vi "TI sbRIO Main (FPGA).vi"() -> ()   [LabVIEW 2013]
uses:
  Type Defs/Controller Names.ctl
  <vilib>/Platform/TimedLoop/XDataNode/timing_clust.ctl
  <vilib>/Platform/TimedLoop/XDataNode/nitl_modes.ctl
  <vilib>/Platform/TimedLoop/XDataNode/wakeup.ctl
  <vilib>/rvi/FXPMathLib/basic elements/FxpIntAccumulator/subVIs/nifxpmath_IntAccumulator_SimConfig.ctl
  <vilib>/rvi/FXPMathLib/FxpSqrt/subVIs/nifxpmath_Sqrt_SimConfig.ctl
  <vilib>/fxp/LVFixedPointOverflowPolicyTypeDef.ctl
  <vilib>/rvi/FXPMathLib/FxpDiv/subVIs/nifxpmath_Div_SimConfig.ctl
  <vilib>/rvi/Emulation/niFpgaSctlEmulationGetInTimedLoop.vi
  <vilib>/rvi/Emulation/niFpgaEmulationReportErrorSimple.vi
  <vilib>/rvi/Emulation/niFpgaGetClockAttributes.vi
  <vilib>/rvi/eio/common/nirviEmuTemplateMethod_errors.vi
  <vilib>/rvi/Emulation/niFpgaCriticalErrorInLSC.vi
  <vilib>/rvi/Analysis/common/codeGenErrors/XNode/niFpgaXNodeCodeGenErrorHandle.vi
  <vilib>/rvi/FXPMathLib/basic elements/FxpIntAccumulator/simVIs/DllFxpIntAccumulator_sub.vi
  <vilib>/rvi/Analysis/utilities/niFPGA Threshold Crossing Logic.vi
  <vilib>/rvi/FXPMathLib/FxpSqrt/simVIs/DllSqrtTemp_sub.vi
  <vilib>/rvi/FXPMathLib/FxpDiv/simVIs/DllFxpDivTemp_sub.vi
  <vilib>/eio/EIONode/EIONode.xnode
  <vilib>/rvi/FXPMathLib/FxpMul/XNode/nifxpmath_Multiplier.xnode
  <vilib>/rvi/FXPMathLib/FxpAdd/XNode/nifxpmath_Add.xnode
  <vilib>/rvi/FXPMathLib/FxpSub/XNode/nifxpmath_Sub.xnode
  <vilib>/rvi/Analysis/measure/period/templates/niFPGA Period Edge Direction.ctl
  <vilib>/rvi/Analysis/measure/mean-var-std/XNode/niFpgaMean-Var-Std.xnode
  <vilib>/Platform/TimedLoop/XDataNode/XDataNode.xnode
  <vilib>/rvi/FXPMathLib/basic elements/FxpIntAccumulator/XNode/nifxpmath_IntAccumulator.xnode
  <vilib>/rvi/Analysis/measure/period/XNode/niFpgaAnalogPeriod.xnode
  <vilib>/rvi/Analysis/measure/dc-rms/XNode/niFpgaDC-RMS.xnode
  <vilib>/rvi/FXPMathLib/FxpSqrt/XNode/nifxpmath_Sqrt.xnode
  <vilib>/rvi/FXPMathLib/FxpDiv/XNode/nifxpmath_Div.xnode
  <vilib>/rvi/FXPMathLib/sim/FxpSim.dll
  <vilib>/Platform/TimedLoop/XDataNode/XDNodeRunTimeDep.lvlib
  <vilib>/rvi/DataTransferAndStorage/Container/XNode/niFpgaContainer.xnode
  <vilib>/rvi/FIFO/Fifo_Resource/niFpgaFifoEmulationRefIn.vi
panel:
  out "Spare_3":fxp<+/-,20,12>
  out "Spare_1":fxp<+/-,20,12>
  in  "Mod1 On?":bool
  in  "Mod2 On?":bool
  in  "Mod2 Pulsing?":bool
  in  "Mod3 Pulsing?":bool
  in  "Mod1 Pulsing?":bool
  in  "Mod3 On?":bool
  in  "Module 3 Pulse Duty":i16
  in  "Module 2 Pulse Duty":i16
  in  "Module 1 Pulse Duty":i16
  in  "Pulse Frequency":sgl=20.0
  in  "Controller Type:":T1
  in  "InvertPWM":bool
  in  "Conti Window":i32=434
  out "Temp 2":fxp<+/-,16,8> format="%#.1f"
  out "Currents (RMS)":fxp<+,26,7>[](array[numeric])
  out "Speed (RPM)":fxp<+,32,18>[](array[numeric])
  in  "Spike Window":i32=125
  in  "Min Window":i32=125
  in  "Max Window":i32=125
  in  "Disarm Level":i32=125
  in  "Arm Level":i32=125
  in  "PS Control":bool=TRUE
  out "Temp":fxp<+/-,16,8> format="%#.1f"
  in  "AO3":fxp<+/-,20,5>
  in  "AO2":fxp<+/-,20,5>
  in  "AO1":fxp<+/-,20,5>
  in  "AO0":fxp<+/-,20,5>
  in  "Kuhnke Window":i32=125
  in  "Speed Hysteresis":fxp<+,23,5>=1.0
  in  "Current Offset":fxp<+/-,18,7>=-60.09521484375 format="%#_14g"
  in  "Current Scale":fxp<+,16,5>=24.0380859375 format="%#_13g"
  out "Actual Loop Time":u32
  in  "Loop Timer (uSec)":u32=100
  in  "Current Offsets":fxp<+/-,24,7>[](array[numeric])=[0.0, 0.0, 0.0, 0.0, 0.0, 0.0]
  out "Elapsed Times":u64[](array[numeric])
  in  "Timer Resets":bool[](array[boolean])=[FALSE, FALSE, FALSE, FALSE, FALSE, FALSE]
  in  "Threshold":fxp<+/-,24,6>=1.0
  in  "Consec Samples":i32=125
  out "Actual Pump Starts":u32[](array[numeric])
  in  "Reset":bool
  in  "Duty (Ticks) 6":i32
  in  "Duty (Ticks) 5":i32
  in  "Duty (Ticks) 4":i32
  in  "Duty (Ticks) 3":i32
  in  "PWM Period (Ticks)":u32=40000000
  in  "Duty (Ticks) 1":i32
  in  "Duty (Ticks) 2":i32
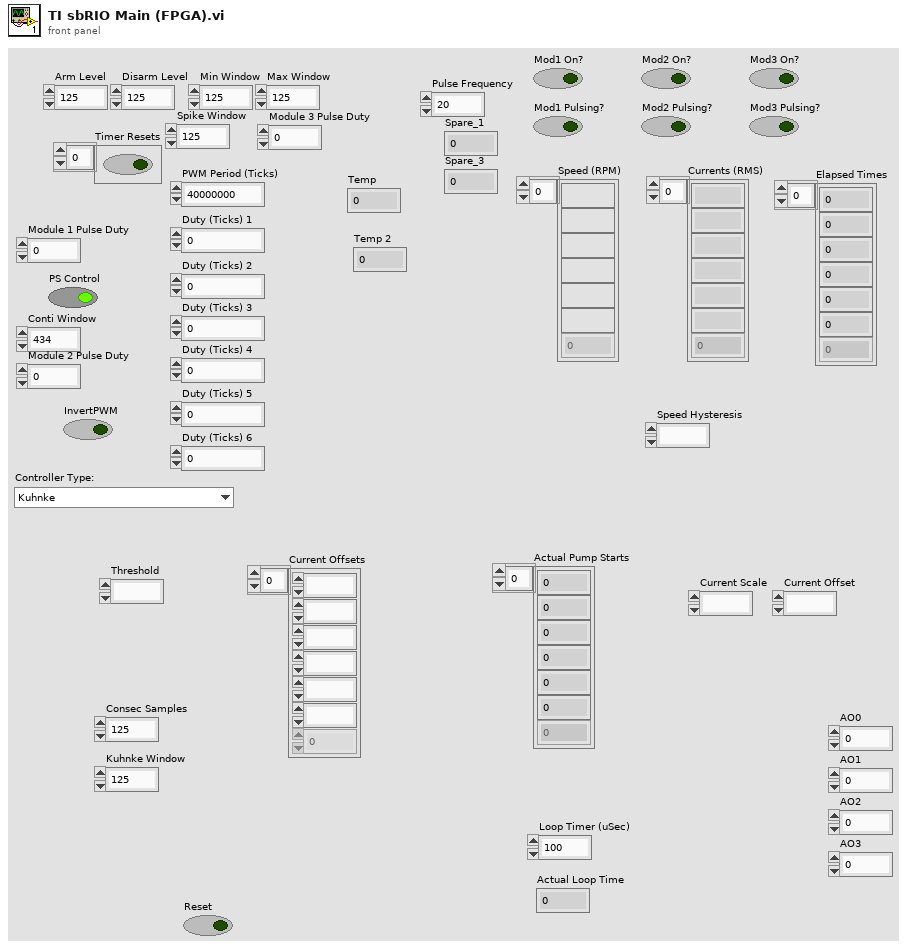
[diagram p1: front panel]
types:
  T1 = typedef "Controller Names.ctl" = enum16{"Kuhnke", "Conti", "Helbako", "TI PWM", "PSA", "Hella Gas", "Hella Diesel", "8 Comm", "10 Comm", "8 Comm Hella", "10 Comm Hella", "8 Comm Omron", "10 Comm Omron", "8 Comm Nissan", "10 Comm Nissan"}
  T2 = typedef "XDNodeRunTimeDep.lvlib/timing_clust.ctl" = cluster{"Expected End [f-1]":u64, "Actual End [f-1]":u64, "Finished Late? [f-1]":bool, "Expected End [i-1]":u64, "Actual End [i-1]":u64, "Finished Late? [i-1]":bool, "Expected Start [i]":u64, "Actual Start [i]":u64, "Expected Start [f]":u64, "Actual Start [f]":u64, "Source Name":string, "Structure Name":string, "Period":i64, "Deadline":i64, "Offset":i64, "Start":i64, "Priority":i32, "Timeout":i32, "Mode":T3, "Wakeup Reason":T4, "Error":errorcluster, "Source Type":string, "Secondary Source Type":string, "Global End Time":u64, "Global Start Time":u64, "Frame Duration":u64, "Iteration Duration":u64, "Assigned CPU":i32, "I/O Scan Engine Mode":u32}
  T3 = typedef "XDNodeRunTimeDep.lvlib/nitl_modes.ctl" = enum32{"No Change", "Process missed periods, maintain original phase", "Discard missed periods, maintain original phase", "Process missed periods, ignore original phase", "Discard missed periods, ignore original phase"}
  T4 = typedef "XDNodeRunTimeDep.lvlib/wakeup.ctl" = enum32{"Normal", "Aborted", "Asynchronous wakeup", "Timing source error", "Timed loop error", "Timeout"}
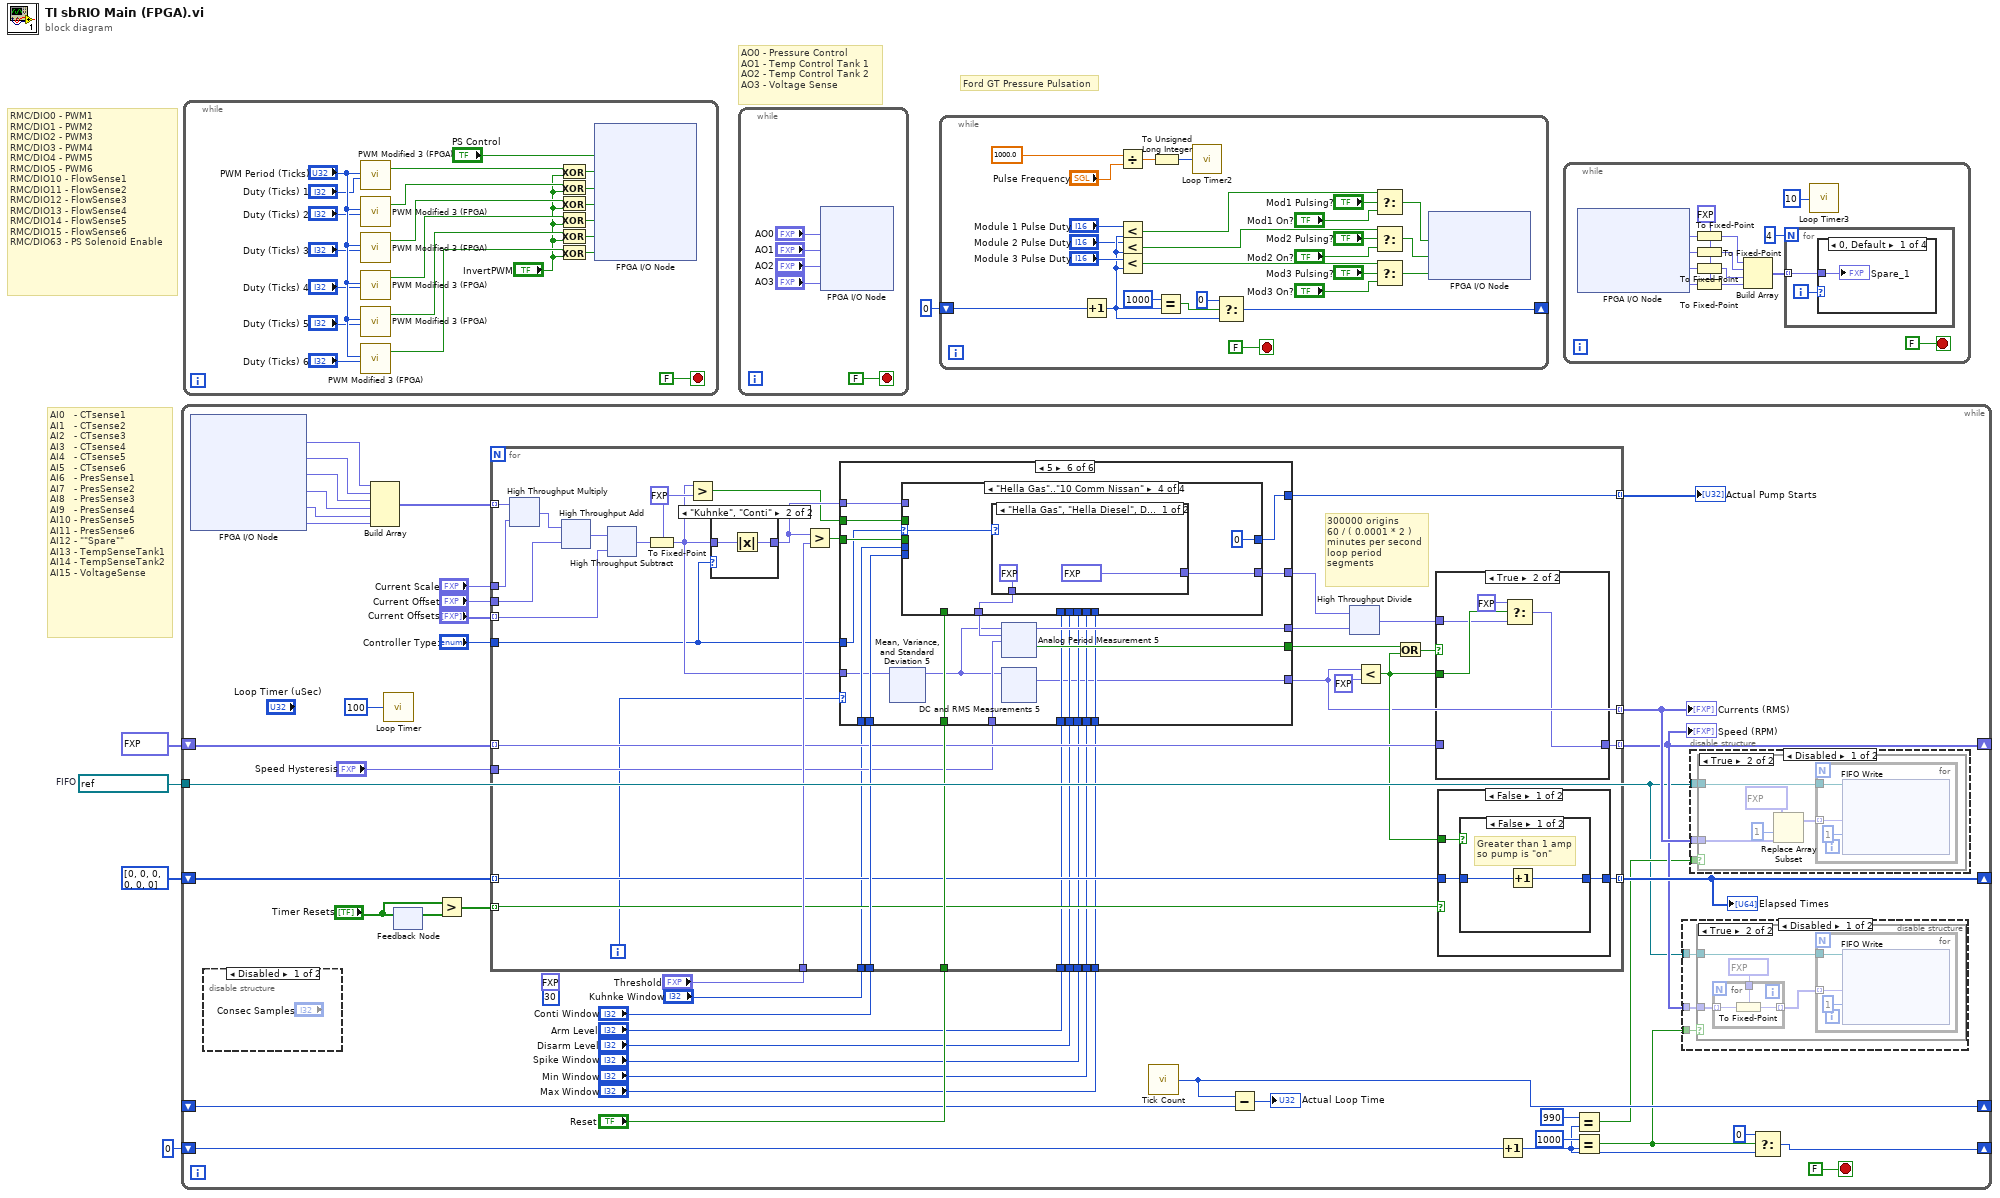
[diagram p0: block diagram]
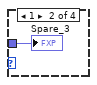
[diagram p2: hidden frame]
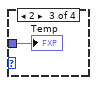
[diagram p3: hidden frame]
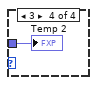
[diagram p4: hidden frame]
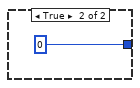
[diagram p12: hidden frame]
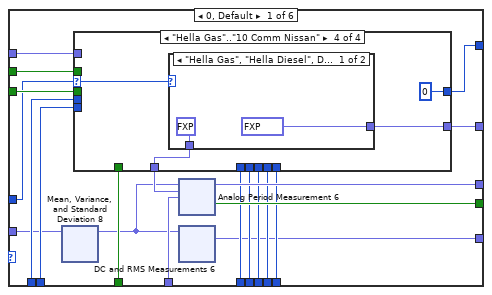
[diagram p14: hidden frame]
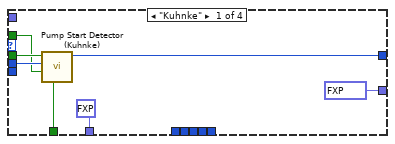
[diagram p15: hidden frame]
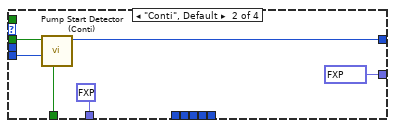
[diagram p16: hidden frame]
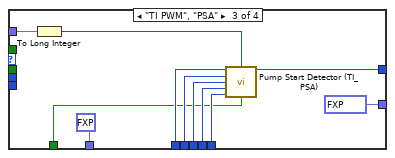
[diagram p17: hidden frame]
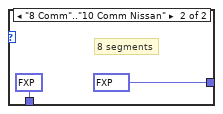
[diagram p18: hidden frame]
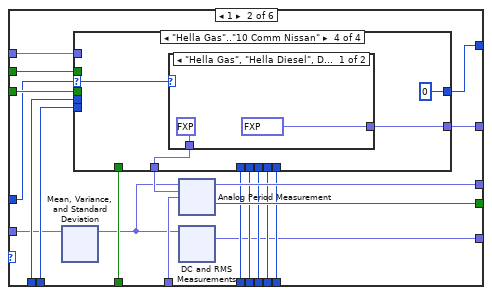
[diagram p19: hidden frame]
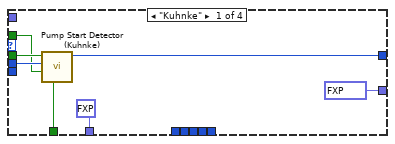
[diagram p20: hidden frame]
diagram:
  w2 = refnum<k21> "Current FIFO"  # FIFO
  # "Ford GT Pressure Pulsation"
  # "RMC/DIO0 - PWM1\nRMC/DIO1 - PWM2\nRMC/DIO2 - PWM3\nRMC/DIO3 - PWM4\nRMC/DIO4 - PWM5\nRMC/DIO5 - PWM6\nRMC/DIO10 - FlowSense1\nRMC/DIO11 - FlowSense2\nRMC/DIO12 - FlowSense3\nRMC/DIO13 - FlowSense4\nRMC/DIO14 - FlowSense5\nRMC/DIO15 - FlowSense6\nRMC/DIO63 - PS Solenoid Enable"
  # "AO0 - Pressure Control\nAO1 - Temp Control Tank 1\nAO2 - Temp Control Tank 2\nAO3 - Voltage Sense"
  # "AI0   - CTsense1\nAI1   - CTsense2\nAI2   - CTsense3\nAI3   - CTsense4\nAI4   - CTsense5\nAI5   - CTsense6\nAI6   - PresSense1\nAI7   - PresSense2\nAI8   - PresSense3\nAI9   - PresSense4\nAI10 - PresSense5\nAI11 - PresSense6\nAI12 - \"\"Spare\"\"\nAI13 - TempSenseTank1\nAI14 - TempSenseTank2\nAI15 - VoltageSense"
  n1 = while {
    shift-right: [w10] -> _
    shift-left: fxp<+,32,18>[] [0.0, 0.0, 0.0, 0.0, 0.0, 0.0] -> [w45]
    shift-right: [w43] -> _
    shift-left: u64[] [0, 0, 0, 0, 0, 0] -> [w44]
    shift-right: [w38] -> _
    shift-left: _ -> [w37]
    shift-right: [w14] -> _
    shift-left: u32 0 ("Tick Count(uSec)") -> [w17]
    tunnel: w2 -> [w7]
    stop <- FALSE stop-if-true
    (unwired) fxp<+/-,24,6> 1.0 ("Threshold")
    (unwired) 30 ("Kuhnke Window")
    n2 = xnode "FPGA I/O Node"() -> ("Current 1 (AI0)"=w28:fxp<+/-,24,5>, "Current 2 (AI1)"=w49:fxp<+/-,24,5>, "Current 3 (AI2)"=w32:fxp<+/-,24,5>, "Current 4 (AI3)"=w31:fxp<+/-,24,5>, "Current 5 (AI4)"=w30:fxp<+/-,24,5>, "Current 6 (AI5)"=w29:fxp<+/-,24,5>)  [unwired: 6 in, 6 out]
    n3 = disable-structure shown="Disabled" {
      frame Disabled {
      }
      frame Enabled {
      }
    }
    n4 = Build Array(w28, w49, w32, w31, w30, w29) -> (w46:fxp<+/-,24,5>[])
    n5 = call "Loop Timer"("Count(uSec)"=u32 100 ("Loop Timer (uSec)")) -> ()  [unwired: 1 out]
    n6 = feedback-in #1("Timer Resets") -> ()
    n7 = feedback #1() -> (w41:bool[])  [unwired: 1 in]
    n8 = Greater?(x="Timer Resets", y=w41) -> (0:w40:bool[])
    n9 = for {
      tunnel: "Conti Window" -> [w111]
      tunnel: [w110] -> w27 mode=indexing
      tunnel: "Threshold" -> [w109]
      tunnel: "Reset" -> [w107]
      tunnel: w46 -> [w91] mode=indexing
      tunnel: w44 -> [w98] mode=indexing
      tunnel: [w97] -> w43 mode=indexing
      tunnel: w45 -> [w102] mode=indexing
      tunnel: [w101] -> w10 mode=indexing
      tunnel: w40 -> [w96] mode=indexing
      tunnel: "Current Offsets" -> [w88] mode=indexing
      tunnel: [w76] -> w13 mode=indexing
      tunnel: "Current Scale" -> [w90]
      tunnel: "Current Offset" -> [w89]
      tunnel: "Speed Hysteresis" -> [w95]
      tunnel: "Kuhnke Window" -> [w94]
      tunnel: "Arm Level" -> [w85]
      tunnel: "Disarm Level" -> [w84]
      tunnel: "Spike Window" -> [w83]
      tunnel: "Min Window" -> [w82]
      tunnel: "Max Window" -> [w81]
      tunnel: "Controller Type:" -> [w74]
      i -> [w77]
      w79 = fxp<+/-,26,7> 0.0 ("out")
      # "300000 origins\n60 / ( 0.0001 * 2 )\nminutes per second\nloop period\nsegments"
      n10 = xnode ("High Throughput Multiply")("x"=w91, "y"=w90) -> ("x*y"=w92:fxp<+/-,40,10>)
      n11 = xnode ("High Throughput Add")("x"=w92, "y"=w89) -> ("x+y"=w80:fxp<+/-,41,11>)
      n12 = xnode "High Throughput Subtract"("x"=w80, "y"=w88) -> ("x-y"=w93:fxp<+/-,42,12>)
      n13 = To Fixed-Point(fixed-point type=w79, number=w93) -> (fixed-point=w75:fxp<+/-,26,7>)
      n14 = Greater?(x=w75, y=w79) -> (0:w78:bool)
      n15 = case shown="\"Kuhnke\", \"Conti\"" w74 {
        tunnel: w75 -> [w112 w113]
        tunnel: [w112 w114] -> w87
        frame Default {
        }
        frame "Kuhnke", "Conti" {
          n16 = Absolute Value(x=w113) -> (abs(x)=w114:fxp<+,26,7>)
        }
      }
      n17 = Greater?(x=w87, y=w109) -> (0:w108:bool)
      n18 = case shown="5" w77 {
        tunnel: w108 -> [w174 w526 w878 w1230 w1582 w1934]
        tunnel: w111 -> [w173 w525 w877 w1229 w1581 w1933]
        tunnel: [w172 w524 w876 w1228 w1580 w1932] -> w110
        tunnel: w107 -> [w166 w518 w870 w1222 w1574 w1926]
        tunnel: w75 -> [w155 w507 w859 w1211 w1563 w1915]
        tunnel: [w157 w509 w861 w1213 w1565 w1917] -> w76
        tunnel: [w171 w523 w875 w1227 w1579 w1931] -> w103
        tunnel: [w170 w522 w874 w1226 w1578 w1930] -> w100
        tunnel: w74 -> [w169 w521 w873 w1225 w1577 w1929]
        tunnel: w95 -> [w168 w520 w872 w1224 w1576 w1928]
        tunnel: w94 -> [w167 w519 w871 w1223 w1575 w1927]
        tunnel: w87 -> [w165 w517 w869 w1221 w1573 w1925]
        tunnel: [w164 w516 w868 w1220 w1572 w1924] -> w86
        tunnel: w85 -> [w163 w515 w867 w1219 w1571 w1923]
        tunnel: w84 -> [w162 w514 w866 w1218 w1570 w1922]
        tunnel: w83 -> [w161 w513 w865 w1217 w1569 w1921]
        tunnel: w82 -> [w160 w512 w864 w1216 w1568 w1920]
        tunnel: w81 -> [w159 w511 w863 w1215 w1567 w1919]
        tunnel: w78 -> [w158 w510 w862 w1214 w1566 w1918]
        frame 0, Default {
          n19 = xnode ("Mean, Variance, and Standard Deviation 8")("input data"=w155) -> ("mean"=w154:fxp<+/-,26,7>)  [unwired: 1 in, 1 out]
          n20 = case shown="\"Hella Gas\"..\"10 Comm Nissan\"" w169 {
            selector: w169 -> [_ _ _ w277]
            tunnel: w174 -> [w256 w263 _ _]
            tunnel: w173 -> [_ w262 _ _]
            tunnel: [w255 w261 w267 u32 0 ("Restarts")] -> w172
            tunnel: w166 -> [w257 w260 w265 _]
            tunnel: w167 -> [w254 _ _ _]
            tunnel: w165 -> [_ _ w274 _]
            tunnel: [fxp<+,32,19> 300000.0 ("x") fxp<+,32,19> 300000.0 ("x") fxp<+,32,19> 300000.0 ("x") w276] -> w164
            tunnel: w163 -> [_ _ w272 _]
            tunnel: w162 -> [_ _ w271 _]
            tunnel: w161 -> [_ _ w270 _]
            tunnel: w160 -> [_ _ w269 _]
            tunnel: w159 -> [_ _ w268 _]
            tunnel: w158 -> [w252 _ _ _]
            tunnel: [fxp<+/-,24,7> 0.0 ("threshold level") fxp<+/-,24,7> 0.0 ("threshold level") fxp<+/-,24,7> 0.0 ("threshold level") w275] -> w156
            frame "Kuhnke" {
              n21 = call "Pump Start Detector (Kuhnke).vi"("Reset"=w257, "Pos?"=w252, "Window"=w254, "Pos Cross"=w256) -> ("Starts"=w255:u32)  [unwired: 6 in, 1 out]
            }
            frame "Conti", Default {
              n22 = call "Pump Start Detector (Conti).vi"("Reset"=w260, "Consec Samples"=w262, "Crossing?"=w263) -> ("Restarts"=w261:u32)  [unwired: 8 in]
            }
            frame "TI PWM", "PSA" {
              n23 = To Long Integer(number=w274) -> (32bit integer=w266:i32)
              n24 = call "Pump Start Detector (TI_PSA).vi"("Arm Level"=w272, "Level"=w266, "Disarm Level"=w271, "Spike Window"=w270, "Min Window"=w269, "Max Window"=w268, "Reset"=w265) -> ("Restarts"=w267:u32)  [unwired: 8 in]
            }
            frame "Hella Gas".."10 Comm Nissan" {
              n25 = case shown="\"Hella Gas\", \"Hella Diesel\", Default" w277 {
                tunnel: [fxp<+,32,19> 300000.0 ("x") fxp<+,32,19> 75000.0 ("x")] -> w276
                tunnel: [fxp<+/-,24,7> 0.0 ("threshold level") fxp<+/-,24,7> 6.75 ("threshold level")] -> w275
                frame "Hella Gas", "Hella Diesel", Default {
                }
                frame "8 Comm".."10 Comm Nissan" {
                  # "8 segments"
                }
              }
            }
          }
          n26 = xnode ("Analog Period Measurement 6")("input data"=w154, "threshold level"=w156, "hysteresis"=w168) -> ("period (samples)"=w170:fxp<+,32,16>, "output valid"=w171:bool)  [unwired: 2 in, 2 out]
          n27 = xnode ("DC and RMS Measurements 6")("input data"=w154) -> ("RMS"=w157:fxp<+,26,7>)  [unwired: 1 in, 1 out]
        }
        frame 1 {
          n28 = xnode ("Mean, Variance, and Standard Deviation")("input data"=w507) -> ("mean"=w506:fxp<+/-,26,7>)  [unwired: 1 in, 1 out]
          n29 = case shown="\"Hella Gas\"..\"10 Comm Nissan\"" w521 {
            selector: w521 -> [_ _ _ w629]
            tunnel: w526 -> [w608 w615 _ _]
            tunnel: w525 -> [_ w614 _ _]
            tunnel: [w607 w613 w619 u32 0 ("Restarts")] -> w524
            tunnel: w518 -> [w609 w612 w617 _]
            tunnel: w519 -> [w606 _ _ _]
            tunnel: w517 -> [_ _ w626 _]
            tunnel: [fxp<+,32,19> 300000.0 ("x") fxp<+,32,19> 300000.0 ("x") fxp<+,32,19> 300000.0 ("x") w628] -> w516
            tunnel: w515 -> [_ _ w624 _]
            tunnel: w514 -> [_ _ w623 _]
            tunnel: w513 -> [_ _ w622 _]
            tunnel: w512 -> [_ _ w621 _]
            tunnel: w511 -> [_ _ w620 _]
            tunnel: w510 -> [w604 _ _ _]
            tunnel: [fxp<+/-,24,7> 0.0 ("threshold level") fxp<+/-,24,7> 0.0 ("threshold level") fxp<+/-,24,7> 0.0 ("threshold level") w627] -> w508
            frame "Kuhnke" {
              n30 = call "Pump Start Detector (Kuhnke).vi"("Reset"=w609, "Pos?"=w604, "Window"=w606, "Pos Cross"=w608) -> ("Starts"=w607:u32)  [unwired: 6 in, 1 out]
            }
            frame "Conti", Default {
              n31 = call "Pump Start Detector (Conti).vi"("Reset"=w612, "Consec Samples"=w614, "Crossing?"=w615) -> ("Restarts"=w613:u32)  [unwired: 8 in]
            }
            frame "TI PWM", "PSA" {
              n32 = To Long Integer(number=w626) -> (32bit integer=w618:i32)
              n33 = call "Pump Start Detector (TI_PSA).vi"("Arm Level"=w624, "Level"=w618, "Disarm Level"=w623, "Spike Window"=w622, "Min Window"=w621, "Max Window"=w620, "Reset"=w617) -> ("Restarts"=w619:u32)  [unwired: 8 in]
            }
            frame "Hella Gas".."10 Comm Nissan" {
              n34 = case shown="\"Hella Gas\", \"Hella Diesel\", Default" w629 {
                tunnel: [fxp<+,32,19> 300000.0 ("x") fxp<+,32,19> 75000.0 ("x")] -> w628
                tunnel: [fxp<+/-,24,7> 0.0 ("threshold level") fxp<+/-,24,7> 6.75 ("threshold level")] -> w627
                frame "Hella Gas", "Hella Diesel", Default {
                }
                frame "8 Comm".."10 Comm Nissan" {
                  # "8 segments"
                }
              }
            }
          }
          n35 = xnode ("Analog Period Measurement")("input data"=w506, "threshold level"=w508, "hysteresis"=w520) -> ("period (samples)"=w522:fxp<+,32,16>, "output valid"=w523:bool)  [unwired: 2 in, 2 out]
          n36 = xnode ("DC and RMS Measurements")("input data"=w506) -> ("RMS"=w509:fxp<+,26,7>)  [unwired: 1 in, 1 out]
        }
        frame 2 {
          n37 = xnode ("Mean, Variance, and Standard Deviation 2")("input data"=w859) -> ("mean"=w858:fxp<+/-,26,7>)  [unwired: 1 in, 1 out]
          n38 = case shown="\"Hella Gas\"..\"10 Comm Nissan\"" w873 {
            selector: w873 -> [_ _ _ w981]
            tunnel: w878 -> [w960 w967 _ _]
            tunnel: w877 -> [_ w966 _ _]
            tunnel: [w959 w965 w971 u32 0 ("Restarts")] -> w876
            tunnel: w870 -> [w961 w964 w969 _]
            tunnel: w871 -> [w958 _ _ _]
            tunnel: w869 -> [_ _ w978 _]
            tunnel: [fxp<+,32,19> 300000.0 ("x") fxp<+,32,19> 300000.0 ("x") fxp<+,32,19> 300000.0 ("x") w980] -> w868
            tunnel: w867 -> [_ _ w976 _]
            tunnel: w866 -> [_ _ w975 _]
            tunnel: w865 -> [_ _ w974 _]
            tunnel: w864 -> [_ _ w973 _]
            tunnel: w863 -> [_ _ w972 _]
            tunnel: w862 -> [w956 _ _ _]
            tunnel: [fxp<+/-,24,7> 0.0 ("threshold level") fxp<+/-,24,7> 0.0 ("threshold level") fxp<+/-,24,7> 0.0 ("threshold level") w979] -> w860
            frame "Kuhnke" {
              n39 = call "Pump Start Detector (Kuhnke).vi"("Reset"=w961, "Pos?"=w956, "Window"=w958, "Pos Cross"=w960) -> ("Starts"=w959:u32)  [unwired: 6 in, 1 out]
            }
            frame "Conti", Default {
              n40 = call "Pump Start Detector (Conti).vi"("Reset"=w964, "Consec Samples"=w966, "Crossing?"=w967) -> ("Restarts"=w965:u32)  [unwired: 8 in]
            }
            frame "TI PWM", "PSA" {
              n41 = To Long Integer(number=w978) -> (32bit integer=w970:i32)
              n42 = call "Pump Start Detector (TI_PSA).vi"("Arm Level"=w976, "Level"=w970, "Disarm Level"=w975, "Spike Window"=w974, "Min Window"=w973, "Max Window"=w972, "Reset"=w969) -> ("Restarts"=w971:u32)  [unwired: 8 in]
            }
            frame "Hella Gas".."10 Comm Nissan" {
              n43 = case shown="\"Hella Gas\", \"Hella Diesel\", Default" w981 {
                tunnel: [fxp<+,32,19> 300000.0 ("x") fxp<+,32,19> 75000.0 ("x")] -> w980
                tunnel: [fxp<+/-,24,7> 0.0 ("threshold level") fxp<+/-,24,7> 6.75 ("threshold level")] -> w979
                frame "Hella Gas", "Hella Diesel", Default {
                }
                frame "8 Comm".."10 Comm Nissan" {
                  # "8 segments"
                }
              }
            }
          }
          n44 = xnode ("Analog Period Measurement 2")("input data"=w858, "threshold level"=w860, "hysteresis"=w872) -> ("period (samples)"=w874:fxp<+,32,16>, "output valid"=w875:bool)  [unwired: 2 in, 2 out]
          n45 = xnode ("DC and RMS Measurements 2")("input data"=w858) -> ("RMS"=w861:fxp<+,26,7>)  [unwired: 1 in, 1 out]
        }
        frame 3 {
          n46 = xnode ("Mean, Variance, and Standard Deviation 3")("input data"=w1211) -> ("mean"=w1210:fxp<+/-,26,7>)  [unwired: 1 in, 1 out]
          n47 = case shown="\"Hella Gas\"..\"10 Comm Nissan\"" w1225 {
            selector: w1225 -> [_ _ _ w1333]
            tunnel: w1230 -> [w1312 w1319 _ _]
            tunnel: w1229 -> [_ w1318 _ _]
            tunnel: [w1311 w1317 w1323 u32 0 ("Restarts")] -> w1228
            tunnel: w1222 -> [w1313 w1316 w1321 _]
            tunnel: w1223 -> [w1310 _ _ _]
            tunnel: w1221 -> [_ _ w1330 _]
            tunnel: [fxp<+,32,19> 300000.0 ("x") fxp<+,32,19> 300000.0 ("x") fxp<+,32,19> 300000.0 ("x") w1332] -> w1220
            tunnel: w1219 -> [_ _ w1328 _]
            tunnel: w1218 -> [_ _ w1327 _]
            tunnel: w1217 -> [_ _ w1326 _]
            tunnel: w1216 -> [_ _ w1325 _]
            tunnel: w1215 -> [_ _ w1324 _]
            tunnel: w1214 -> [w1308 _ _ _]
            tunnel: [fxp<+/-,24,7> 0.0 ("threshold level") fxp<+/-,24,7> 0.0 ("threshold level") fxp<+/-,24,7> 0.0 ("threshold level") w1331] -> w1212
            frame "Kuhnke" {
              n48 = call "Pump Start Detector (Kuhnke).vi"("Reset"=w1313, "Pos?"=w1308, "Window"=w1310, "Pos Cross"=w1312) -> ("Starts"=w1311:u32)  [unwired: 6 in, 1 out]
            }
            frame "Conti", Default {
              n49 = call "Pump Start Detector (Conti).vi"("Reset"=w1316, "Consec Samples"=w1318, "Crossing?"=w1319) -> ("Restarts"=w1317:u32)  [unwired: 8 in]
            }
            frame "TI PWM", "PSA" {
              n50 = To Long Integer(number=w1330) -> (32bit integer=w1322:i32)
              n51 = call "Pump Start Detector (TI_PSA).vi"("Arm Level"=w1328, "Level"=w1322, "Disarm Level"=w1327, "Spike Window"=w1326, "Min Window"=w1325, "Max Window"=w1324, "Reset"=w1321) -> ("Restarts"=w1323:u32)  [unwired: 8 in]
            }
            frame "Hella Gas".."10 Comm Nissan" {
              n52 = case shown="\"Hella Gas\", \"Hella Diesel\", Default" w1333 {
                tunnel: [fxp<+,32,19> 300000.0 ("x") fxp<+,32,19> 75000.0 ("x")] -> w1332
                tunnel: [fxp<+/-,24,7> 0.0 ("threshold level") fxp<+/-,24,7> 6.75 ("threshold level")] -> w1331
                frame "Hella Gas", "Hella Diesel", Default {
                }
                frame "8 Comm".."10 Comm Nissan" {
                  # "8 segments"
                }
              }
            }
          }
          n53 = xnode ("Analog Period Measurement 3")("input data"=w1210, "threshold level"=w1212, "hysteresis"=w1224) -> ("period (samples)"=w1226:fxp<+,32,16>, "output valid"=w1227:bool)  [unwired: 2 in, 2 out]
          n54 = xnode ("DC and RMS Measurements 3")("input data"=w1210) -> ("RMS"=w1213:fxp<+,26,7>)  [unwired: 1 in, 1 out]
        }
        frame 4 {
          n55 = xnode ("Mean, Variance, and Standard Deviation 4")("input data"=w1563) -> ("mean"=w1562:fxp<+/-,26,7>)  [unwired: 1 in, 1 out]
          n56 = case shown="\"Hella Gas\"..\"10 Comm Nissan\"" w1577 {
            selector: w1577 -> [_ _ _ w1685]
            tunnel: w1582 -> [w1664 w1671 _ _]
            tunnel: w1581 -> [_ w1670 _ _]
            tunnel: [w1663 w1669 w1675 u32 0 ("Restarts")] -> w1580
            tunnel: w1574 -> [w1665 w1668 w1673 _]
            tunnel: w1575 -> [w1662 _ _ _]
            tunnel: w1573 -> [_ _ w1682 _]
            tunnel: [fxp<+,32,19> 300000.0 ("x") fxp<+,32,19> 300000.0 ("x") fxp<+,32,19> 300000.0 ("x") w1684] -> w1572
            tunnel: w1571 -> [_ _ w1680 _]
            tunnel: w1570 -> [_ _ w1679 _]
            tunnel: w1569 -> [_ _ w1678 _]
            tunnel: w1568 -> [_ _ w1677 _]
            tunnel: w1567 -> [_ _ w1676 _]
            tunnel: w1566 -> [w1660 _ _ _]
            tunnel: [fxp<+/-,24,7> 0.0 ("threshold level") fxp<+/-,24,7> 0.0 ("threshold level") fxp<+/-,24,7> 0.0 ("threshold level") w1683] -> w1564
            frame "Kuhnke" {
              n57 = call "Pump Start Detector (Kuhnke).vi"("Reset"=w1665, "Pos?"=w1660, "Window"=w1662, "Pos Cross"=w1664) -> ("Starts"=w1663:u32)  [unwired: 6 in, 1 out]
            }
            frame "Conti", Default {
              n58 = call "Pump Start Detector (Conti).vi"("Reset"=w1668, "Consec Samples"=w1670, "Crossing?"=w1671) -> ("Restarts"=w1669:u32)  [unwired: 8 in]
            }
            frame "TI PWM", "PSA" {
              n59 = To Long Integer(number=w1682) -> (32bit integer=w1674:i32)
              n60 = call "Pump Start Detector (TI_PSA).vi"("Arm Level"=w1680, "Level"=w1674, "Disarm Level"=w1679, "Spike Window"=w1678, "Min Window"=w1677, "Max Window"=w1676, "Reset"=w1673) -> ("Restarts"=w1675:u32)  [unwired: 8 in]
            }
            frame "Hella Gas".."10 Comm Nissan" {
              n61 = case shown="\"Hella Gas\", \"Hella Diesel\", Default" w1685 {
                tunnel: [fxp<+,32,19> 300000.0 ("x") fxp<+,32,19> 75000.0 ("x")] -> w1684
                tunnel: [fxp<+/-,24,7> 0.0 ("threshold level") fxp<+/-,24,7> 6.75 ("threshold level")] -> w1683
                frame "Hella Gas", "Hella Diesel", Default {
                }
                frame "8 Comm".."10 Comm Nissan" {
                  # "8 segments"
                }
              }
            }
          }
          n62 = xnode ("Analog Period Measurement 4")("input data"=w1562, "threshold level"=w1564, "hysteresis"=w1576) -> ("period (samples)"=w1578:fxp<+,32,16>, "output valid"=w1579:bool)  [unwired: 2 in, 2 out]
          n63 = xnode ("DC and RMS Measurements 4")("input data"=w1562) -> ("RMS"=w1565:fxp<+,26,7>)  [unwired: 1 in, 1 out]
        }
        frame 5 {
          n64 = xnode ("Mean, Variance, and Standard Deviation 5")("input data"=w1915) -> ("mean"=w1914:fxp<+/-,26,7>)  [unwired: 1 in, 1 out]
          n65 = case shown="\"Hella Gas\"..\"10 Comm Nissan\"" w1929 {
            selector: w1929 -> [_ _ _ w2037]
            tunnel: w1934 -> [w2016 w2023 _ _]
            tunnel: w1933 -> [_ w2022 _ _]
            tunnel: [w2015 w2021 w2027 u32 0 ("Restarts")] -> w1932
            tunnel: w1926 -> [w2017 w2020 w2025 _]
            tunnel: w1927 -> [w2014 _ _ _]
            tunnel: w1925 -> [_ _ w2034 _]
            tunnel: [fxp<+,32,19> 300000.0 ("x") fxp<+,32,19> 300000.0 ("x") fxp<+,32,19> 300000.0 ("x") w2036] -> w1924
            tunnel: w1923 -> [_ _ w2032 _]
            tunnel: w1922 -> [_ _ w2031 _]
            tunnel: w1921 -> [_ _ w2030 _]
            tunnel: w1920 -> [_ _ w2029 _]
            tunnel: w1919 -> [_ _ w2028 _]
            tunnel: w1918 -> [w2012 _ _ _]
            tunnel: [fxp<+/-,24,7> 0.0 ("threshold level") fxp<+/-,24,7> 0.0 ("threshold level") fxp<+/-,24,7> 0.0 ("threshold level") w2035] -> w1916
            frame "Kuhnke" {
              n66 = call "Pump Start Detector (Kuhnke).vi"("Reset"=w2017, "Pos?"=w2012, "Window"=w2014, "Pos Cross"=w2016) -> ("Starts"=w2015:u32)  [unwired: 6 in, 1 out]
            }
            frame "Conti", Default {
              n67 = call "Pump Start Detector (Conti).vi"("Reset"=w2020, "Consec Samples"=w2022, "Crossing?"=w2023) -> ("Restarts"=w2021:u32)  [unwired: 8 in]
            }
            frame "TI PWM", "PSA" {
              n68 = To Long Integer(number=w2034) -> (32bit integer=w2026:i32)
              n69 = call "Pump Start Detector (TI_PSA).vi"("Arm Level"=w2032, "Level"=w2026, "Disarm Level"=w2031, "Spike Window"=w2030, "Min Window"=w2029, "Max Window"=w2028, "Reset"=w2025) -> ("Restarts"=w2027:u32)  [unwired: 8 in]
            }
            frame "Hella Gas".."10 Comm Nissan" {
              n70 = case shown="\"Hella Gas\", \"Hella Diesel\", Default" w2037 {
                tunnel: [fxp<+,32,19> 300000.0 ("x") fxp<+,32,19> 75000.0 ("x")] -> w2036
                tunnel: [fxp<+/-,24,7> 0.0 ("threshold level") fxp<+/-,24,7> 6.75 ("threshold level")] -> w2035
                frame "Hella Gas", "Hella Diesel", Default {
                }
                frame "8 Comm".."10 Comm Nissan" {
                  # "8 segments"
                }
              }
            }
          }
          n71 = xnode ("Analog Period Measurement 5")("input data"=w1914, "threshold level"=w1916, "hysteresis"=w1928) -> ("period (samples)"=w1930:fxp<+,32,16>, "output valid"=w1931:bool)  [unwired: 2 in, 2 out]
          n72 = xnode ("DC and RMS Measurements 5")("input data"=w1914) -> ("RMS"=w1917:fxp<+,26,7>)  [unwired: 1 in, 1 out]
        }
      }
      n73 = xnode "High Throughput Divide"("x"=w86, "y"=w100) -> ("x/y"=w104:fxp<+,32,18>)
      n74 = Less?(x=w76, y=fxp<+,24,6> 1.0 ("current threshold")) -> (x < y?=w99:bool)
      n75 = Or(x=w103, y=w99) -> (x .or. y?=w105:bool)
      n76 = case shown="True" w105 {
        tunnel: w104 -> [_ w124]
        tunnel: w99 -> [_ w125]
        tunnel: w102 -> [w122 _]
        tunnel: [w122 w123] -> w101
        frame False {
        }
        frame True {
          n77 = Select(t=fxp<+,32,18> 0.0 ("input data"), s=w125, f=w124) -> (s? t:f=w123:fxp<+,32,18>)
        }
      }
      n78 = case shown="False" w96 {
        tunnel: w99 -> [w117 _]
        tunnel: w98 -> [w116 _]
        tunnel: [w115 u64 0] -> w97
        frame False {
          n79 = case shown="False" w117 {
            tunnel: w116 -> [w119 w120]
            tunnel: [w118 w120] -> w115
            frame False {
              # "Greater than 1 amp\nso pump is \"on\""
              n80 = Increment(x=w119) -> (x+1=w118:u64)
            }
            frame True {
            }
          }
        }
        frame True {
        }
      }
    }
    "Actual Pump Starts" <- w27
    "Elapsed Times" <- w43
    "Speed (RPM)" <- w10
    "Currents (RMS)" <- w13
    n81 = call "Tick Count"() -> ("Tick Count(uSec)"=w38:u32)
    n82 = Subtract(x=w38, y=w37) -> (x-y=→"Actual Loop Time":u32)
    n83 = Increment(x=w17) -> (x+1=w12:u32)
    n84 = Equal?(x=u32 990, y=w12) -> (x = y?=w9:bool)
    n85 = Equal?(x=u32 1000, y=w12) -> (x = y?=w8:bool)
    n86 = disable-structure shown="Disabled" {
      disable-tunnel: w10 -> [w63 _]
      disable-tunnel: w8 -> [w62 _]
      disable-tunnel: w7 -> [w61 _]
      frame Disabled {
        n87 = case shown="True" w62 {
          tunnel: w61 -> [_ w67]
          tunnel: w63 -> [_ w65]
          frame False {
          }
          frame True {
            n88 = for {
              tunnel: fxp<+/-,35,16> -32768.0 ("Element") -> [w70]
              tunnel: w65 -> [w69] mode=indexing
              tunnel: [w68] -> w64 mode=indexing
              n89 = To Fixed-Point(fixed-point type=w70, number=w69) -> (fixed-point=w68:fxp<+/-,35,16>)
            }
            n90 = for {
              tunnel: w67 -> [w73]
              tunnel: w64 -> [w71] mode=indexing
              n91 = xnode ("FIFO Write")("Element"=w71, "Timeout"=1, "FIFO In"=w73) -> ()  [unwired: 2 out]
            }
          }
        }
      }
      frame Enabled {
      }
    }
    n92 = disable-structure shown="Disabled" {
      disable-tunnel: w13 -> [w52 _]
      disable-tunnel: w9 -> [w51 _]
      disable-tunnel: w7 -> [w50 _]
      frame Disabled {
        n93 = case shown="True" w51 {
          tunnel: w50 -> [_ w57]
          tunnel: w52 -> [_ w56]
          frame False {
          }
          frame True {
            n94 = Replace Array Subset(array=fxp<+/-,35,16>[] [-32768.0, -32768.0, -32768.0, -32768.0, -32768.0, -32768.0, -32768.0], new element=w56, index=1) -> (w54:fxp<+/-,35,16>[])
            n95 = for {
              tunnel: w57 -> [w60]
              tunnel: w54 -> [w58] mode=indexing
              n96 = xnode ("FIFO Write")("Element"=w58, "Timeout"=1, "FIFO In"=w60) -> ()  [unwired: 2 out]
            }
          }
        }
      }
      frame Enabled {
      }
    }
    n97 = Select(t=u32 0 ("x"), s=w8, f=w12) -> (s? t:f=w14:u32)
  }
  n98 = while {
    stop <- FALSE stop-if-true
    n99 = call "PWM Modified 3 (FPGA).vi"("PWM Period (Ticks)"="PWM Period (Ticks)", "PWM Duty Cycle (Ticks)"="Duty (Ticks) 1") -> ("PWM DO"=w2273:bool)  [unwired: 14 in, 3 out]
    n100 = call "PWM Modified 3 (FPGA).vi"("PWM Period (Ticks)"="PWM Period (Ticks)", "PWM Duty Cycle (Ticks)"="Duty (Ticks) 2") -> ("PWM DO"=w2274:bool)  [unwired: 14 in, 3 out]
    n101 = call "PWM Modified 3 (FPGA).vi"("PWM Period (Ticks)"="PWM Period (Ticks)", "PWM Duty Cycle (Ticks)"="Duty (Ticks) 3") -> ("PWM DO"=w2275:bool)  [unwired: 14 in, 3 out]
    n102 = call "PWM Modified 3 (FPGA).vi"("PWM Period (Ticks)"="PWM Period (Ticks)", "PWM Duty Cycle (Ticks)"="Duty (Ticks) 4") -> ("PWM DO"=w2276:bool)  [unwired: 14 in, 3 out]
    n103 = call "PWM Modified 3 (FPGA).vi"("PWM Period (Ticks)"="PWM Period (Ticks)", "PWM Duty Cycle (Ticks)"="Duty (Ticks) 5") -> ("PWM DO"=w2277:bool)  [unwired: 14 in, 3 out]
    n104 = call "PWM Modified 3 (FPGA).vi"("PWM Period (Ticks)"="PWM Period (Ticks)", "PWM Duty Cycle (Ticks)"="Duty (Ticks) 6") -> ("PWM DO"=w2278:bool)  [unwired: 14 in, 3 out]
    n105 = Exclusive Or(1:"InvertPWM", 2:w2273) -> (0:w2272:bool)
    n106 = Exclusive Or(1:"InvertPWM", 2:w2274) -> (0:w2271:bool)
    n107 = Exclusive Or(1:"InvertPWM", 2:w2275) -> (0:w2270:bool)
    n108 = Exclusive Or(1:"InvertPWM", 2:w2276) -> (0:w2269:bool)
    n109 = Exclusive Or(1:"InvertPWM", 2:w2277) -> (0:w2268:bool)
    n110 = Exclusive Or(1:"InvertPWM", 2:w2278) -> (0:w2267:bool)
    n111 = xnode "FPGA I/O Node"("RMC/DIO63"="PS Control", "RMC/DIO0"=w2272, "RMC/DIO1"=w2271, "RMC/DIO2"=w2270, "RMC/DIO3"=w2269, "RMC/DIO4"=w2268, "RMC/DIO5"=w2267) -> ()  [unwired: 8 in, 8 out]
  }
  n112 = while {
    stop <- FALSE stop-if-true
    n113 = xnode "FPGA I/O Node"("AO0"="AO0", "AO1"="AO1", "AO2"="AO2", "AO3"="AO3") -> ()  [unwired: 4 in, 4 out]
  }
  n114 = while {
    shift-right: [w2308] -> _
    shift-left: i16 0 -> [w2313]
    stop <- FALSE stop-if-true
    n115 = Increment(x=w2313) -> (x+1=w2307:i16)
    n116 = Divide(x=sgl 1000.0, y="Pulse Frequency") -> (x/y=w2315:sgl)
    n117 = Less?(x="Module 1 Pulse Duty", y=w2307) -> (x < y?=w2296:bool)
    n118 = Less?(x="Module 2 Pulse Duty", y=w2307) -> (x < y?=w2297:bool)
    n119 = Less?(x="Module 3 Pulse Duty", y=w2307) -> (x < y?=w2298:bool)
    n120 = To Unsigned Long Integer(number=w2315) -> (unsigned 32bit integer=w2314:u32)
    n121 = Equal?(x=i16 1000, y=w2307) -> (x = y?=w2311:bool)
    n122 = call "Loop Timer2"("Count(uSec)"=w2314) -> ()  [unwired: 1 out]
    n123 = Select(t=i16 0, s=w2311, f=w2307) -> (s? t:f=w2308:i16)
    n124 = Select(t=w2296, s="Mod1 Pulsing?", f="Mod1 On?") -> (s? t:f=w2293:bool)
    n125 = Select(t=w2297, s="Mod2 Pulsing?", f="Mod2 On?") -> (s? t:f=w2294:bool)
    n126 = Select(t=w2298, s="Mod3 Pulsing?", f="Mod3 On?") -> (s? t:f=w2295:bool)
    n127 = xnode "FPGA I/O Node"("RMC/DIO15"=w2293, "RMC/DIO31"=w2294, "RMC/DIO47"=w2295) -> ()  [unwired: 3 in, 3 out]
  }
  n128 = while {
    stop <- FALSE stop-if-true
    w2321 = fxp<+/-,16,8> 0.0
    n129 = xnode "FPGA I/O Node"() -> ("Spare_1"=w2322:fxp<+/-,24,5>, "Spare_3"=w2323:fxp<+/-,24,5>, "Temp 1 (AI13)"=w2329:fxp<+/-,24,5>, "Temp 2 (AI14)"=w2327:fxp<+/-,24,5>)  [unwired: 4 in, 4 out]
    n130 = To Fixed-Point(fixed-point type=w2321, number=w2322) -> (fixed-point=w2319:fxp<+/-,16,8>)
    n131 = To Fixed-Point(fixed-point type=w2321, number=w2323) -> (fixed-point=w2320:fxp<+/-,16,8>)
    n132 = To Fixed-Point(fixed-point type=w2321, number=w2329) -> (fixed-point=w2328:fxp<+/-,16,8>)
    n133 = To Fixed-Point(fixed-point type=w2321, number=w2327) -> (fixed-point=w2326:fxp<+/-,16,8>)
    n134 = Build Array(w2319, w2320, w2328, w2326) -> (w2325:fxp<+/-,16,8>[])
    n135 = for {
      N: 4 -> [_]
      tunnel: w2325 -> [w2332] mode=indexing
      i -> [w2333]
      n136 = case shown="0, Default" w2333 {
        tunnel: w2332 -> [w2334 w2335 w2336 w2337]
        frame 0, Default {
          "Spare_1" <- w2334
        }
        frame 1 {
          "Spare_3" <- w2335
        }
        frame 2 {
          "Temp" <- w2336
        }
        frame 3 {
          "Temp 2" <- w2337
        }
      }
    }
    n137 = call "Loop Timer3"("Count(mSec)"=u32 10 ("Count(uSec)")) -> ()  [unwired: 1 out]
  }
